vi "IncSteps.vi"(1 "I/O chan for motion end":i32=2, 2 "1-D (F) 2-D (T)":bool, 3 "wait time between scans (ms)":i32, 4 "Steps to move":i32=100, 5 "Axis":i32=1 min=1 max=4, 6 "number of scans":i32=128, 7 "I/O chan for motor pulse":i32=7) -> (0 "Output String":string)   [LabVIEW 2022 SP3]
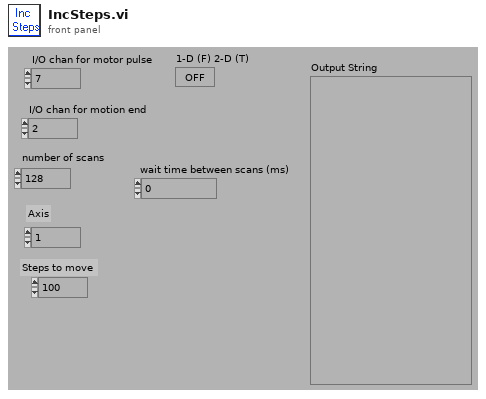
[diagram p1: front panel]
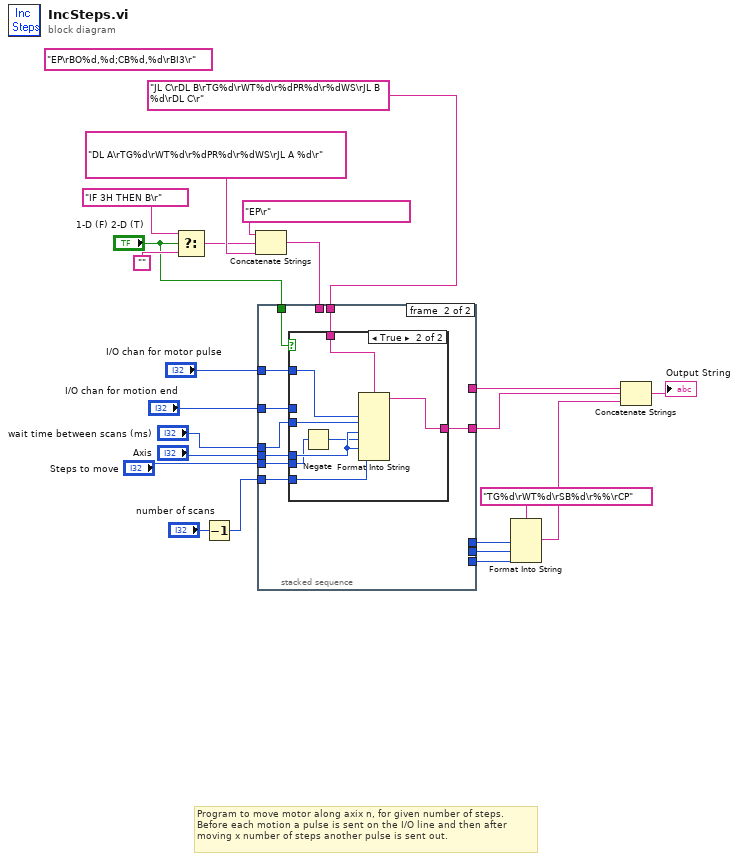
[diagram p0: block diagram]
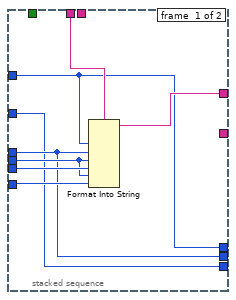
[diagram p2: hidden frame]
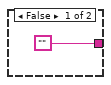
[diagram p3: hidden frame]
diagram:
  (unwired) "EP\rBO%d,%d;CB%d,%d\rBI3\r"
  # "Program to move motor along axix n, for given number of steps.\nBefore each motion a pulse is sent on the I/O line and then after\nmoving x number of steps another pulse is sent out."
  n1 = Select(t="IF 3H THEN B\r" ("f"), s="1-D (F) 2-D (T)", f="") -> (s? t:f=w13:string)
  n2 = Decrement(x="number of scans") -> (x-1=w19:i32)
  n3 = Concatenate Strings("EP\r", w13, "DL A\rTG%d\rWT%d\r%dPR%d\r%dWS\rJL A %d\r") -> (w12:string)
  n4 = stacked-sequence {
    tunnel: [w31 _] -> w5
    tunnel: "Steps to move" -> [w30 w35]
    tunnel: "Axis" -> [w29 w36]
    tunnel: w19 -> [w28 w37]
    tunnel: "wait time between scans (ms)" -> [w26 w34]
    tunnel: "I/O chan for motor pulse" -> [w25 w39]
    tunnel: "I/O chan for motion end" -> [w24 w38]
    tunnel: w12 -> [w27 _]
    tunnel: "1-D (F) 2-D (T)" -> [_ w40]
    tunnel: [w24 _] -> w8
    tunnel: [w26 _] -> w7
    tunnel: [w25 _] -> w6
    tunnel: [_ w33] -> w2
    tunnel: "JL C\rDL B\rTG%d\rWT%d\r%dPR%d\r%dWS\rJL B %d\rDL C\r" -> [_ w32]
    frame #0 {
      n5 = Format Into String(format string=w27, w25, w26, w29, w30, w29, w28) -> (resulting string=w31:string)  [unwired: 2 in, 1 out]
    }
    frame #1 {
      n6 = case shown="True" w40 {
        tunnel: w39 -> [_ w42]
        tunnel: w38 -> [_ _]
        tunnel: w37 -> [_ w49]
        tunnel: w36 -> [_ w48]
        tunnel: w35 -> [_ w47]
        tunnel: w34 -> [_ w45]
        tunnel: ["" w44] -> w33
        tunnel: w32 -> [_ w43]
        frame False {
        }
        frame True {
          n7 = Negate(x=w47) -> (-x=w46:i32)
          n8 = Format Into String(format string=w43, w42, w45, w48, w46, w48, w49) -> (resulting string=w44:string)  [unwired: 2 in, 1 out]
        }
      }
    }
  }
  n9 = Format Into String(format string="TG%d\rWT%d\rSB%d\r%%\rCP", w6, w7, w8) -> (resulting string=w4:string)  [unwired: 2 in, 1 out]
  n10 = Concatenate Strings(w5, w2, w4) -> (→"Output String":string)
